vi "Fuel Injector Analysis Selection.vi"(8 "error in (no error)":errorcluster, 11 "Node Ptr":T3 format="%.0x") -> (0 "error out":errorcluster)   [LabVIEW 2015, in "Fuel Injection Addon System Explorer.lvlib"]
uses:
  Fuel Injection Addon System Explorer.lvlib
  <vilib>/NI Veristand/Custom Device API/Custom Device Item Ref.ctl
  Shared/Types/Stage.PullIn.Types.ctl
  Shared/Types/Stage.Transition.Types.ctl
  <vilib>/NI Veristand/Custom Device API/Custom Device Channel.ctl
  <vilib>/NI Veristand/Custom Device API/Custom Device Channel Type.ctl
  Types/Stage.Settings.ctl
  Shared/Constants.vi
  <vilib>/NI Veristand/Custom Device Tools/Custom Device Utility Library/NI VeriStand - Search for All Items by GUID.vi
  <vilib>/NI VeriStand/Custom Device API/Custom Device API.lvlib
  <vilib>/NI Veristand/Custom Device Tools/Custom Device Utility Library/Custom Device Utility Library.lvlib
  Shared/Fuel Injection Addon Shared.lvlib
panel:
  in  "Stage.Level":dbl
  in  "PullIn.Level":dbl=1.0
  in  "Stage.Transition":T1
  in  "PullIn.Type":T2
  in  "Analysis":i32(listbox)=7
  in  "Reset":bool
  in  "Apply":bool
  in  "SHDocVw.IWebBrowser":refnum<k7>(container)
  in  "Header":cluster{"Section Name":string}={"Section Name"="Custom Device Item Settings"}
  in  "Description":string
  out "Name":string
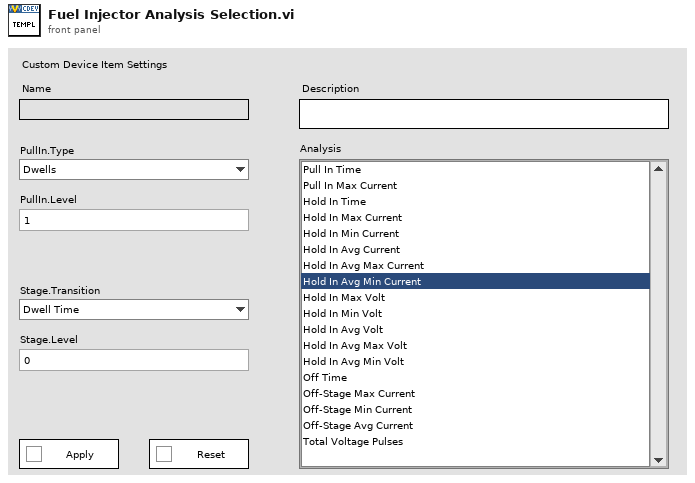
[diagram p1: front panel]
types:
  T1 = typedef "Stage.Transition.Types.ctl" = enum8{"Dwell Time", "Voltage Level"}
  T2 = typedef "Stage.PullIn.Types.ctl" = enum8{"Dwells", "Current Drop"}
  T3 = typedef "Custom Device API.lvlib/Custom Device Item Ref.ctl" = u64
  T4 = typedef "Custom Device API.lvlib/Custom Device Item Info.ctl" = cluster{"Name":string, "Is Channel":bool, "GUID":string, "Is Waveform":bool}
  T5 = typedef "Fuel Injection Addon Shared.lvlib/Analysis.Channels.Select.ctl" = cluster{"Pull In Time":bool, "Pull In Max Current":bool, "Hold In Time":bool, "Hold In Max Current":bool, "Hold In Min Current":bool, "Hold In Avg Current":bool, "Hold In Avg Max Current":bool, "Hold In Avg Min Current":bool, "Hold In Max Volt":bool, "Hold In Min Volt":bool, "Hold In Avg Volt":bool, "Hold In Avg Max Volt":bool, "Hold In Avg Min Volt":bool, "Off Time":bool, "Off-Stage Max Current":bool, "Off-Stage Min Current":bool, "Off-Stage Avg Current":bool, "Total Voltage Pulses":bool}
  T6 = typedef "Fuel Injection Addon System Explorer.lvlib/Stage.Settings.ctl" = cluster{"PullIn.Type":T2, "Stage.Transition":T1}
  T7 = typedef "Custom Device API.lvlib/Custom Device Commands.ctl" = enum16{"Default", "Item renamed", "Shutdown", "Dynamic button pressed"}
  T8 = typedef "Custom Device API.lvlib/Custom Device Channel.ctl" = cluster{"Type":T9, "Units":string, "Default Value":dbl, "Faultable":bool, "Scalable":bool}
  T9 = typedef "Custom Device API.lvlib/Custom Device Channel Type.ctl" = enum16{"Input", "Output"}
  T10 = typedef "LVPoint32TypeDef.ctl" = cluster{"Horizontal":i32, "Vertical":i32}
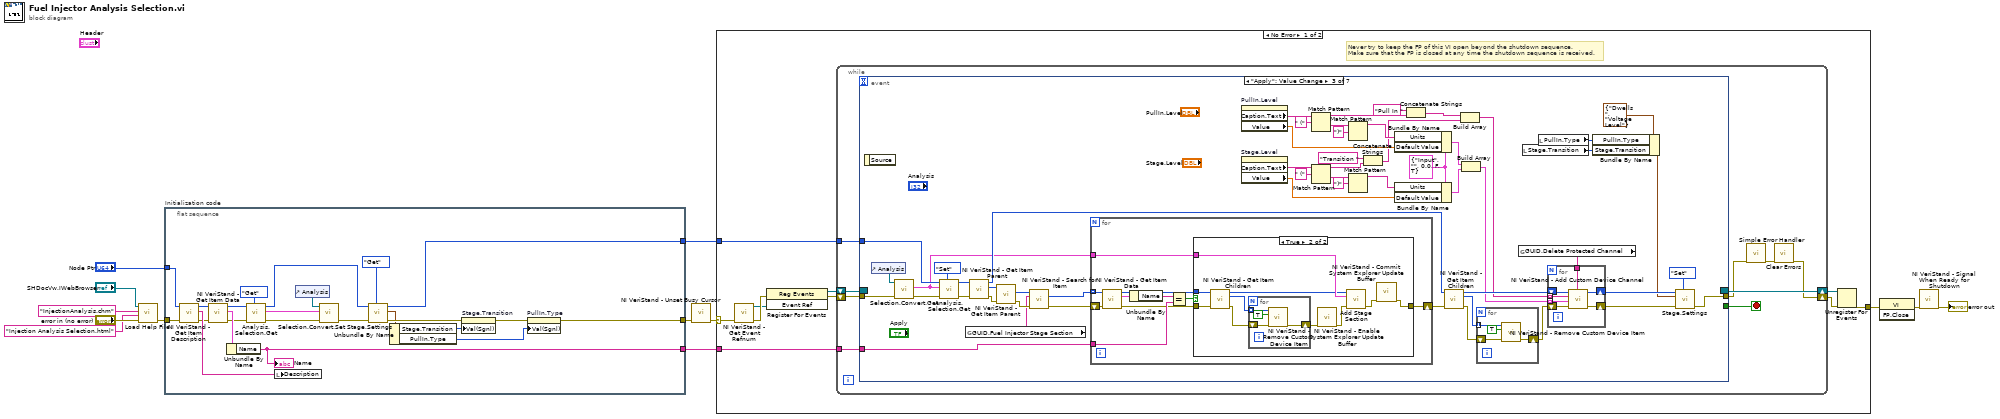
[diagram p0: block diagram]
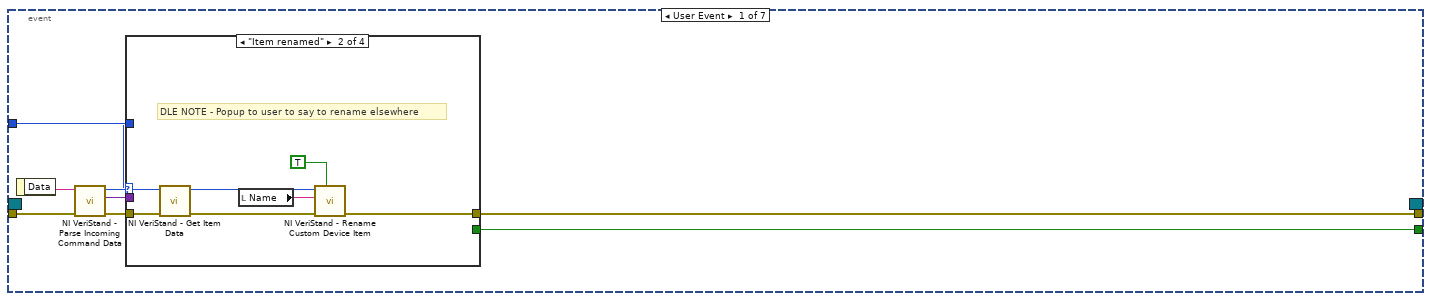
[diagram p2: hidden frame]
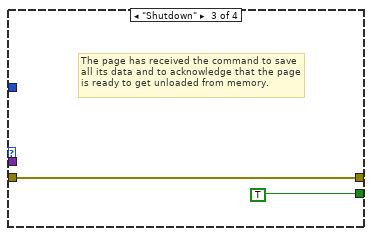
[diagram p4: hidden frame]
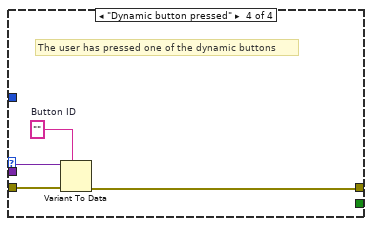
[diagram p5: hidden frame]
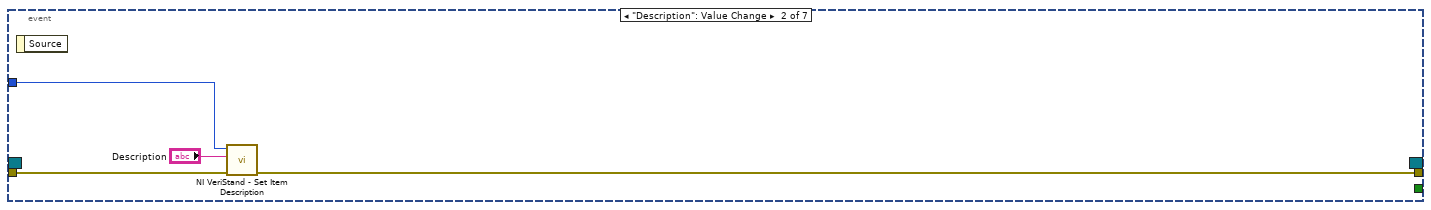
[diagram p6: hidden frame]
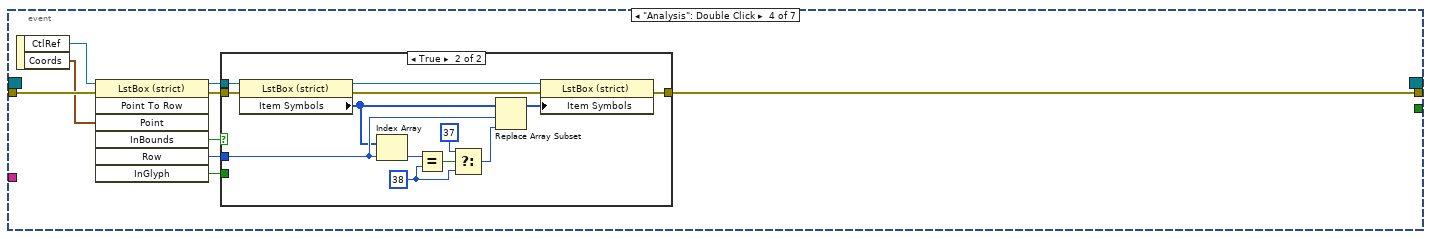
[diagram p8: hidden frame]
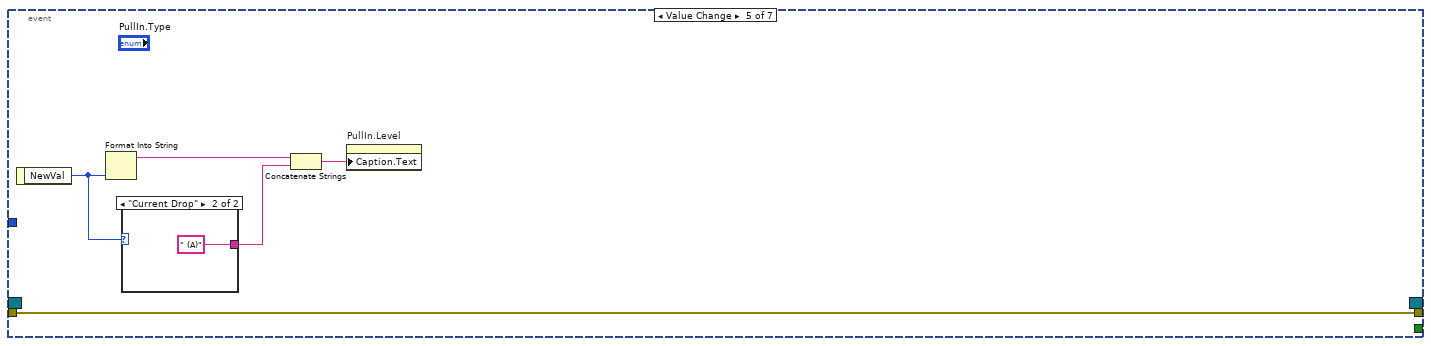
[diagram p10: hidden frame]
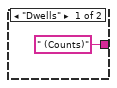
[diagram p11: hidden frame]
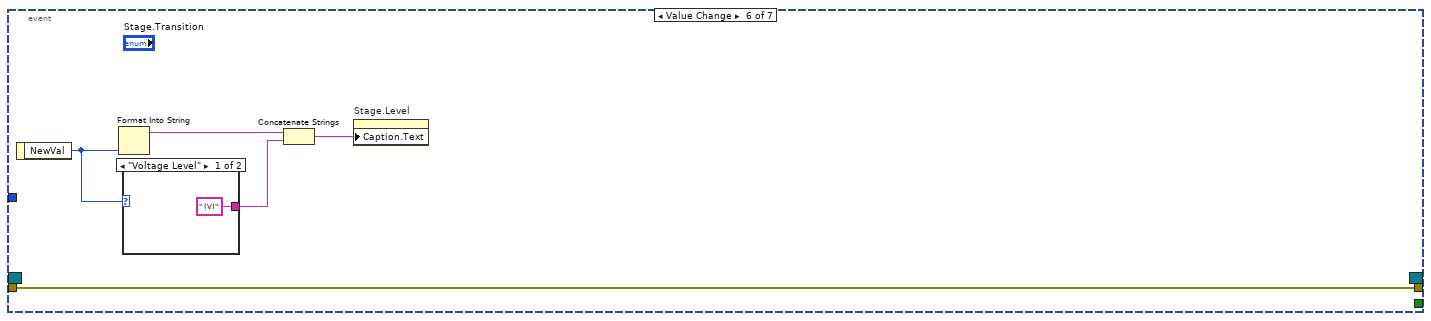
[diagram p12: hidden frame]
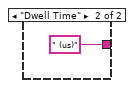
[diagram p13: hidden frame]
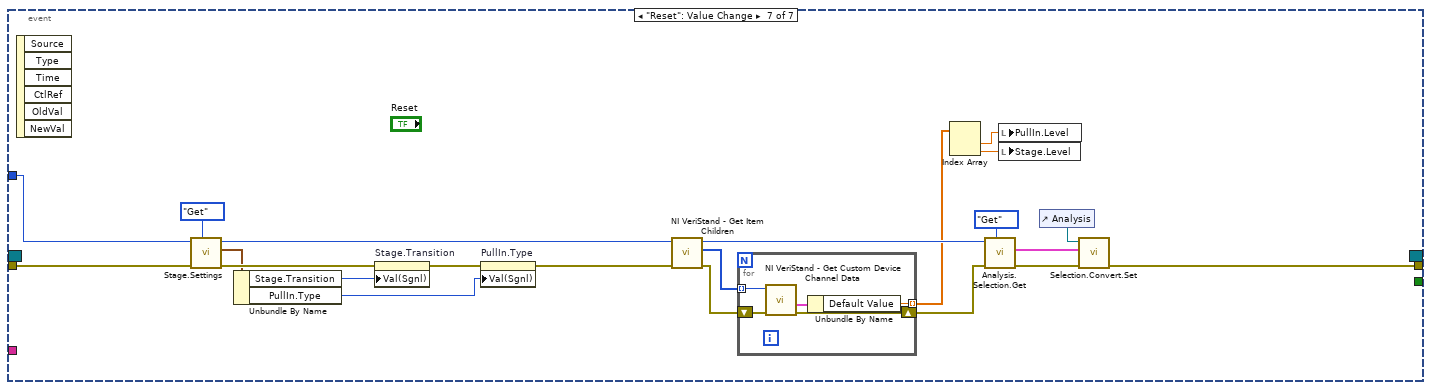
[diagram p14: hidden frame]
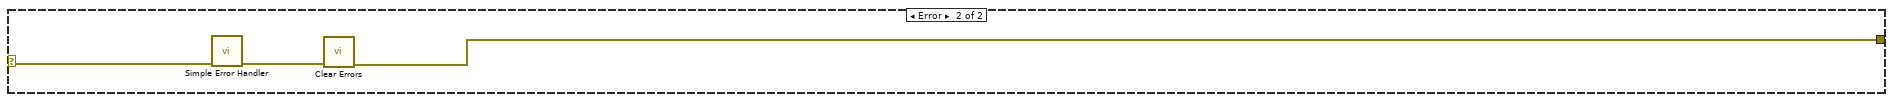
[diagram p15: hidden frame]
diagram:
  n1 = call "Load Help File.vi"("error in (no error)"="error in (no error)", "HTML File"="Injection Analysis Selection.html" ("Main CHM File"), "Main CHM File"="InjectionAnalysis.chm", "SHDocVw.IWebBrowser2"="SHDocVw.IWebBrowser") -> ("error out"=w5:errorcluster)  [unwired: 7 in]
  n2 = flat-sequence "Initialization code" {
    tunnel: w5 -> [w35]
    tunnel: [w15] -> w10
    tunnel: [w17] -> w8
    tunnel: "Node Ptr" -> [w31]
    tunnel: [w28] -> w1
    frame #0 {
      n3 = call <vilib>:"NI VeriStand - Get Item Description.vi"("error in (no error)"=w35, "Item Ref in"=w31) -> ("error out"=w33:errorcluster, "Description"=w34:string, "Item Ref out"=w36:T3)  [unwired: 7 out]
      n4 = call <vilib>:"NI VeriStand - Get Item Data.vi"("error in (no error)"=w33, "Item Ref in"=w36) -> ("error out"=w30:errorcluster, "Item Info"=w32:T4, "Item Ref out"=w29:T3)  [unwired: 7 out]
      n5 = Unbundle By Name(w32) -> ("Name"=w28:string)
      "Name" <- w28
      n6 = call "Analysis.Selection.Get.vi"("Action"=enum8{"Get", "Set"}."Get", "error in (no error)"=w30, "Item Ref in"=w29) -> ("error out"=w25:errorcluster, "Selections"=w26:T5, "Item Ref out"=w14:T3)  [unwired: 6 in]
      n7 = local write "Description"(w34) -> ()
      n8 = control-ref of="Analysis"() -> (w24:refnum<vi>)
      n9 = call "Selection.Convert.Set.vi"("error in (no error)"=w25, "Selections"=w26, "ListBox in"=w24) -> ("error out"=w16:errorcluster)  [unwired: 8 in]
      n10 = call "Stage.Settings.vi"("Action"=enum8{"Get", "Set"}."Get", "error in (no error)"=w16, "Item Ref in"=w14) -> ("error out"=w23:errorcluster, "Settings"=w20:T6, "Item Ref out"=w17:T3)  [unwired: 6 in]
      n11 = Unbundle By Name(w20) -> ("Stage.Transition"=w18:T1, "PullIn.Type"=w19:T2)
      n12 = property on="Stage.Transition" class="Enum (strict)"(error in=w23, "Val(Sgnl)"=w18) -> (error out=w22:errorcluster)  [unwired: 1 in, 1 out]
      n13 = property on="PullIn.Type" class="Enum (strict)"(error in=w22, "Val(Sgnl)"=w19) -> (error out=w15:errorcluster)  [unwired: 1 in, 1 out]
    }
  }
  n14 = call <vilib>:"NI VeriStand - Unset Busy Cursor.vi"("error in (no error)"=w10) -> ("error out"=w9:errorcluster)  [unwired: 10 out]
  n15 = case shown="No Error" w9 {
    selector: w9 -> [w38 w238]
    tunnel: [w43 w236] -> w13
    tunnel: w8 -> [w39 _]
    tunnel: w1 -> [w37 _]
    frame No Error {
      # "Never try to keep the FP of this VI open beyond the shutdown sequence.\nMake sure that the FP is closed at any time the shutdown sequence is received."
      n16 = call <vilib>:"NI VeriStand - Get Event Refnum.vi"("error in (no error)"=w38) -> ("error out"=w46:errorcluster, "Event Ref"=w42:refnum<user-event>)  [unwired: 9 out]
      n17 = register-events(error in=w46, w42) -> (reference out=w40:refnum<event-registration>, error out=w41:errorcluster)  [unwired: 1 in]
      n18 = while {
        tunnel: w39 -> [w51]
        shift-right: [w48] -> w44
        shift-left: w41 -> [w54]
        shift-right: [w55] -> w45
        shift-left: w40 -> [w53]
        tunnel: w37 -> [w47]
        stop <- w52 stop-if-true
        n19 = event shown="[2] \"Apply\": Value Change" {
          selector: w53 -> [_ _ _ _ _ _ _]
          dyn-events: [_ _ _ _ _ _ _] -> w55
          timeout: _ -> [_ _ _ _ _ _ _]
          tunnel: w54 -> [w63 w80 w112 w174 w199 w205 w225]
          tunnel: [w59 _ _ _ _ _ _] -> w52
          tunnel: [w58 w79 w91 w172 w199 w205 w227] -> w50
          tunnel: w51 -> [w57 w81 w126 _ _ _ w224]
          tunnel: w47 -> [_ _ w129 _ _ _ _]
          event User Event {
            n20 = event-data() -> ("Data"=w62:string)  [unwired: 1 out]
            n21 = call <vilib>:"NI VeriStand - Parse Incoming Command Data.vi"("error in (no error)"=w63, "Incoming data"=w62) -> ("error out"=w61:errorcluster, "Outgoing data"=w56:variant, "Action"=w60:T7)  [unwired: 7 out]
            n22 = case shown="\"Item renamed\"" w60 {
              tunnel: w61 -> [w64 w71 w72 w77]
              tunnel: [_ _ TRUE _] -> w59
              tunnel: [w64 w68 w72 w74] -> w58
              tunnel: w57 -> [_ w70 _ _]
              tunnel: w56 -> [_ _ _ w76]
              frame "Default", Default {
              }
              frame "Item renamed" {
                # "DLE NOTE - Popup to user to say to rename elsewhere"
                n23 = call <vilib>:"NI VeriStand - Get Item Data.vi"("error in (no error)"=w71, "Item Ref in"=w70) -> ("error out"=w69:errorcluster, "Item Ref out"=w67:T3)  [unwired: 8 out]
                n24 = local read "Name"() -> (w66:string)
                n25 = call <vilib>:"NI VeriStand - Rename Custom Device Item.vi"("Force Rename (F)"=TRUE, "error in (no error)"=w69, "New Name"=w66, "Item Ref in"=w67) -> ("error out"=w68:errorcluster)  [unwired: 5 in, 2 out]
              }
              frame "Shutdown" {
                # "The page has received the command to save all its data and to acknowledge that the page is ready to get unloaded from memory."
              }
              frame "Dynamic button pressed" {
                w75 = ""  # Button ID
                # "The user has pressed one of the dynamic buttons"
                n26 = Variant To Data(error in=w77, type=w75, Variant=w76) -> (error out=w74:errorcluster)  [unwired: 1 out]
              }
            }
          }
          event "Description": Value Change {
            n27 = event-data() -> ()  [unwired: 2 out]
            n28 = call <vilib>:"NI VeriStand - Set Item Description.vi"("error in (no error)"=w80, "Description"="Description", "Item Ref in"=w81) -> ("error out"=w79:errorcluster)  [unwired: 8 out]
          }
          event "Apply": Value Change {
            w117 = T8 {"Type"=enum."Input", "Units"="", "Default Value"=0.0, "Faultable"=FALSE, "Scalable"=TRUE} ("Channel")
            n29 = event-data() -> ()  [unwired: 2 out]
            n30 = control-ref of="Analysis"() -> (w109:refnum<vi>)
            n31 = call "Selection.Convert.Get.vi"("error in (no error)"=w112, "ListBox in"=w109) -> ("error out"=w111:errorcluster, "Analysis Options"=w110:T5)  [unwired: 8 in]
            n32 = call "Analysis.Selection.Get.vi"("Action"=enum8{"Get", "Set"}."Set", "error in (no error)"=w111, "Selections"=w110, "Item Ref in"=w126) -> ("error out"=w124:errorcluster, "Item Ref out"=w125:T3)  [unwired: 5 in, 1 out]
            n33 = global read "Constants.vi" "GUID.Fuel Injector Stage Section"() -> (w131:string)
            n34 = call <vilib>:"NI VeriStand - Get Item Parent.vi"("error in (no error)"=w124, "Item Ref in"=w125) -> ("error out"=w134:errorcluster, "Parent Ref"=w135:T3, "Item Ref out"=w122:T3)  [unwired: 6 in, 1 out]
            n35 = call <vilib>:"NI VeriStand - Get Item Parent.vi"("error in (no error)"=w134, "Item Ref in"=w135) -> ("error out"=w132:errorcluster, "Parent Ref"=w133:T3)  [unwired: 6 in, 2 out]
            n36 = call-poly <vilib>:"NI VeriStand - Search for Item.vi"("error in"=w132, "Item GUID"=w131, "Section Ref in"=w133) -> ("error out"=w128:errorcluster, "Item Refs"=w130:T3[])  [unwired: 5 in, 2 out]
            n37 = for {
              tunnel: w130 -> [w155] mode=indexing
              shift-right: [w147] -> w123
              shift-left: w128 -> [w156]
              tunnel: w129 -> [w151]
              tunnel: w110 -> [w149]
              n38 = call <vilib>:"NI VeriStand - Get Item Data.vi"("error in (no error)"=w156, "Item Ref in"=w155) -> ("error out"=w148:errorcluster, "Item Info"=w153:T4, "Item Ref out"=w154:T3)  [unwired: 6 in, 1 out]
              n39 = Unbundle By Name(w153) -> ("Name"=w152:string)
              n40 = Equal?(x=w152, y=w151) -> (x = y?=w150:bool)
              n41 = case shown="True" w150 {
                tunnel: [w157 w161] -> w147
                tunnel: w154 -> [_ w167]
                tunnel: w149 -> [_ w166]
                tunnel: w148 -> [w157 w158]
                frame False {
                }
                frame True {
                  n42 = call <vilib>:"NI VeriStand - Get Item Children.vi"("error in (no error)"=w158, "Item Ref in"=w167) -> ("error out"=w163:errorcluster, "Child Refs"=w164:T3[], "Item Ref out"=w165:T3)  [unwired: 6 in, 1 out]
                  n43 = for {
                    tunnel: w164 -> [w171] mode=indexing
                    shift-right: [w169] -> w160
                    shift-left: w163 -> [w170]
                    n44 = call <vilib>:"NI VeriStand - Remove Custom Device Item.vi"("error in (no error)"=w170, "Force Delete (F)"=TRUE, "Item Ref in"=w171) -> ("error out"=w169:errorcluster)  [unwired: 7 in, 1 out]
                  }
                  n45 = call <vilib>:"NI VeriStand - Enable System Explorer Update Buffer.vi"("error in (no error)"=w160) -> ("error out"=w159:errorcluster)  [unwired: 10 in]
                  n46 = call "Add Stage Section.vi"("error in (no error)"=w159, "Analysis Options"=w166, "Shot Section reference in"=w165) -> ("error out"=w162:errorcluster)  [unwired: 7 in, 1 out]
                  n47 = call <vilib>:"NI VeriStand - Commit System Explorer Update Buffer.vi"("error in (no error)"=w162) -> ("error out"=w161:errorcluster)  [unwired: 10 in]
                }
              }
            }
            n48 = property on="PullIn.Level" class="DigNum (strict)"() -> ("Caption.Text"=w97:string, "Value"=w95:dbl)  [unwired: 2 in, 2 out]
            n49 = property on="Stage.Level" class="DigNum (strict)"() -> ("Caption.Text"=w98:string, "Value"=w99:dbl)  [unwired: 2 in, 2 out]
            n50 = Match Pattern(string=w97, regular expression=" (") -> (before substring=w96:string, after substring=w106:string)  [unwired: 1 in, 2 out]
            n51 = Match Pattern(string=w98, regular expression=" (") -> (before substring=w83:string, after substring=w102:string)  [unwired: 1 in, 2 out]
            n52 = Match Pattern(string=w106, regular expression=")") -> (before substring=w104:string)  [unwired: 1 in, 3 out]
            n53 = Match Pattern(string=w102, regular expression=")") -> (before substring=w100:string)  [unwired: 1 in, 3 out]
            n54 = Concatenate Strings("Transition " ("string"), w83) -> (w82:string)
            n55 = Bundle By Name(cluster=w117, "Units"=w104, "Default Value"=w95) -> (w116:T8)
            n56 = Bundle By Name(cluster=w117, "Units"=w100, "Default Value"=w99) -> (w115:T8)
            n57 = Concatenate Strings("Pull In " ("string"), w96) -> (w86:string)
            n58 = call <vilib>:"NI VeriStand - Get Item Children.vi"("error in (no error)"=w123, "Item Ref in"=w122) -> ("error out"=w119:errorcluster, "Child Refs"=w120:T3[], "Item Ref out"=w121:T3)  [unwired: 6 in, 1 out]
            n59 = Build Array(w86, w82) -> (w108:string[])
            n60 = Build Array(w116, w115) -> (w114:T8[])
            n61 = for {
              tunnel: w120 -> [w138] mode=indexing
              shift-right: [w136] -> w118
              shift-left: w119 -> [w137]
              n62 = call <vilib>:"NI VeriStand - Remove Custom Device Item.vi"("error in (no error)"=w137, "Force Delete (F)"=TRUE, "Item Ref in"=w138) -> ("error out"=w136:errorcluster)  [unwired: 7 in, 1 out]
            }
            n63 = global read "Constants.vi" "GUID.Delete Protected Channel"() -> (w113:string)
            n64 = local read "Stage.Transition"() -> (w87:T1)
            n65 = local read "PullIn.Type"() -> (w88:T2)
            n66 = for {
              shift-right: [w145] -> w92
              shift-left: w118 -> [w146]
              tunnel: w114 -> [w143] mode=indexing
              tunnel: w113 -> [w142]
              tunnel: w108 -> [w141] mode=indexing
              shift-right: [w140] -> w93
              shift-left: w121 -> [w144]
              n67 = call <vilib>:"NI VeriStand - Add Custom Device Channel.vi"("GUID (Default Channel)"=w142, "error in (no error)"=w146, "Channel"=w143, "Channel Name"=w141, "Parent Ref in"=w144) -> ("error out"=w145:errorcluster, "Parent Ref out"=w140:T3)  [unwired: 3 in, 2 out]
            }
            n68 = Bundle By Name(cluster=T6 {"PullIn.Type"=enum."Dwells", "Stage.Transition"=enum."Voltage Level"} ("Settings"), "PullIn.Type"=w88, "Stage.Transition"=w87) -> (w89:T6)
            n69 = call "Stage.Settings.vi"("Action"=enum8{"Get", "Set"}."Set", "error in (no error)"=w92, "Settings"=w89, "Item Ref in"=w93) -> ("error out"=w91:errorcluster)  [unwired: 5 in, 2 out]
          }
          event "Analysis": Double Click {
            n70 = event-data() -> ("CtlRef"=w175:refnum<vi>, "Coords"=w173:T10)  [unwired: 1 out]
            n71 = invoke class="LstBox (strict)" method="Point To Row"(reference=w175, error in=w174, "Point"=w173) -> (reference out=w179:refnum<vi>, error out=w178:errorcluster, "InBounds"=w176:bool, "Row"=w177:i32, "InGlyph"=w180:bool)  [unwired: 4 in, 2 out]
            n72 = case shown="True" w176 {
              tunnel: w180 -> [_ _]
              tunnel: w179 -> [_ w194]
              tunnel: w178 -> [w181 w193]
              tunnel: w177 -> [_ w192]
              tunnel: [w181 w182] -> w172
              frame False {
              }
              frame True {
                w189 = 38
                n73 = property class="LstBox (strict)"(reference=w194, error in=w193) -> (reference out=w185:refnum<vi>, error out=w184:errorcluster, "Item Symbols"=w187:i32[])
                n74 = Index Array(array=w187, index=w192) -> (element=w191:i32)
                n75 = Equal?(x=w191, y=w189) -> (x = y?=w190:bool)
                n76 = Select(t=37, s=w190, f=w189) -> (s? t:f=w186:i32)
                n77 = Replace Array Subset(array=w187, new element=w186, index=w192) -> (w183:i32[])
                n78 = property class="LstBox (strict)"(reference=w185, error in=w184, "Item Symbols"=w183) -> (error out=w182:errorcluster)  [unwired: 1 out]
              }
            }
          }
          event Value Change {
            n79 = event-data() -> ("NewVal"=w198:T2)  [unwired: 1 out]
            n80 = Format Into String(w198) -> (resulting string=w196:string)  [unwired: 3 in, 1 out]
            n81 = case shown="\"Current Drop\"" w198 {
              tunnel: [" (Counts)" " (A)"] -> w197
              frame "Dwells" {
              }
              frame "Current Drop" {
              }
            }
            n82 = Concatenate Strings(w196, w197) -> (w195:string)
            n83 = property on="PullIn.Level" class="DigNum (strict)"("Caption.Text"=w195) -> ()  [unwired: 2 in, 2 out]
          }
          event Value Change {
            n84 = event-data() -> ("NewVal"=w204:T1)  [unwired: 1 out]
            n85 = Format Into String(w204) -> (resulting string=w206:string)  [unwired: 3 in, 1 out]
            n86 = case shown="\"Voltage Level\"" w204 {
              tunnel: [" (V)" " (us)"] -> w202
              frame "Voltage Level" {
              }
              frame "Dwell Time" {
              }
            }
            n87 = Concatenate Strings(w206, w202) -> (w203:string)
            n88 = property on="Stage.Level" class="DigNum (strict)"("Caption.Text"=w203) -> ()  [unwired: 2 in, 2 out]
          }
          event "Reset": Value Change {
            n89 = event-data() -> ()  [unwired: 7 out]
            n90 = call "Stage.Settings.vi"("Action"=enum8{"Get", "Set"}."Get", "error in (no error)"=w225, "Item Ref in"=w224) -> ("error out"=w223:errorcluster, "Settings"=w211:T6, "Item Ref out"=w222:T3)  [unwired: 6 in]
            n91 = Unbundle By Name(w211) -> ("Stage.Transition"=w209:T1, "PullIn.Type"=w210:T2)
            n92 = property on="Stage.Transition" class="Enum (strict)"(error in=w223, "Val(Sgnl)"=w209) -> (error out=w214:errorcluster)  [unwired: 1 in, 1 out]
            n93 = property on="PullIn.Type" class="Enum (strict)"(error in=w214, "Val(Sgnl)"=w210) -> (error out=w213:errorcluster)  [unwired: 1 in, 1 out]
            n94 = call <vilib>:"NI VeriStand - Get Item Children.vi"("error in (no error)"=w213, "Item Ref in"=w222) -> ("error out"=w220:errorcluster, "Child Refs"=w219:T3[], "Item Ref out"=w221:T3)  [unwired: 6 in, 1 out]
            n95 = for {
              tunnel: w219 -> [w234] mode=indexing
              tunnel: [w232] -> w217 mode=indexing
              shift-right: [w231] -> w218
              shift-left: w220 -> [w235]
              n96 = call <vilib>:"NI VeriStand - Get Custom Device Channel Data.vi"("error in (no error)"=w235, "Channel Ref in"=w234) -> ("error out"=w231:errorcluster, "Channel"=w233:T8)  [unwired: 4 in, 4 out]
              n97 = Unbundle By Name(w233) -> ("Default Value"=w232:dbl)
            }
            n98 = Index Array(array=w217) -> (element #1=w216:dbl, element #2=w215:dbl)  [unwired: 2 in]
            n99 = call "Analysis.Selection.Get.vi"("Action"=enum8{"Get", "Set"}."Get", "error in (no error)"=w218, "Item Ref in"=w221) -> ("error out"=w228:errorcluster, "Selections"=w226:T5)  [unwired: 6 in, 1 out]
            n100 = local write "PullIn.Level"(w216) -> ()
            n101 = local write "Stage.Level"(w215) -> ()
            n102 = control-ref of="Analysis"() -> (w229:refnum<vi>)
            n103 = call "Selection.Convert.Set.vi"("error in (no error)"=w228, "Selections"=w226, "ListBox in"=w229) -> ("error out"=w227:errorcluster)  [unwired: 8 in]
          }
        }
        n104 = call <vilib>:"Simple Error Handler.vi"("error in (no error)"=w50) -> ("error out"=w49:errorcluster)  [unwired: 1 in, 7 out]
        n105 = call <vilib>:"Clear Errors.vi"("error in (no error)"=w49) -> ("error out"=w48:errorcluster)  [unwired: 1 in, 5 out]
      }
      n106 = Unregister For Events(event registration refnum=w45, error in=w44) -> (error out=w43:errorcluster)
    }
    frame Error {
      n107 = call <vilib>:"Simple Error Handler.vi"("error in (no error)"=w238) -> ("error out"=w237:errorcluster)  [unwired: 1 in, 7 out]
      n108 = call <vilib>:"Clear Errors.vi"("error in (no error)"=w237) -> ("error out"=w236:errorcluster)  [unwired: 1 in, 5 out]
    }
  }
  n109 = invoke class="VI" method="FP.Close"(error in=w13) -> (error out=w12:errorcluster)  [unwired: 2 in, 2 out]
  n110 = call <vilib>:"NI VeriStand - Signal When Ready for Shutdown.vi"("error in (no error)"=w12) -> ("error out"=→"error out":errorcluster)  [unwired: 10 out]
